vi "PXIe 4113 Update Channels.vi"(8 "error in (no error)":errorcluster, 10 "Array":dbl[](array[numeric]), 11 "Resource name in":refnum<k15>) -> (0 "error out":errorcluster, 3 "Resource name out":refnum<k15>)   [LabVIEW 2014, in "PXIe 4113 Engine.lvlib"]
uses:
  PXIe 4113 Engine.lvlib
  <instrlib>/niDCPower/nidcpower.llb/niDCPower Wait For Event - Event.ctl
  <vilib>/NI Veristand/Custom Device Tools/Custom Device Utility Library/Custom Device Utility Library.lvlib
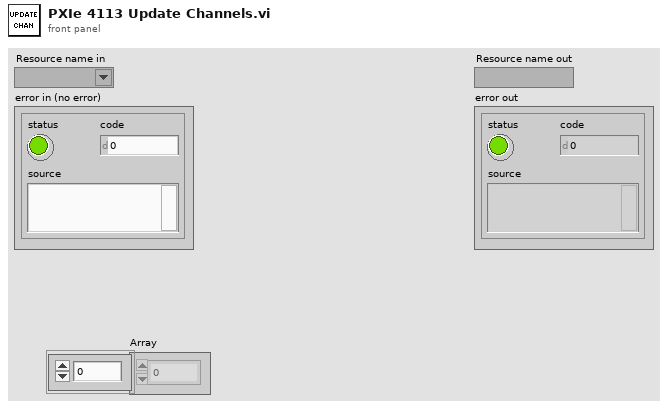
[diagram p1: front panel]
types:
  T1 = typedef "niDCPower Wait For Event - Event.ctl" = i32
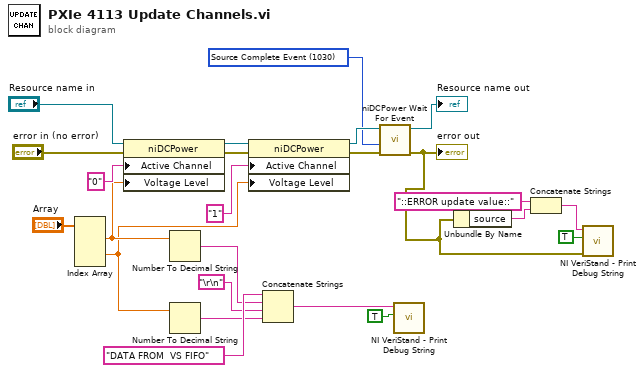
[diagram p0: block diagram]
diagram:
  w15 = T1 1030 items=["Source Complete Event"=1030, "Measure Complete Event"=1031, "Sequence Iteration Complete Event"=1032, "Sequence Engine Done Event"=1033, "Pulse Complete Event"=1051, "Ready For Pulse Trigger Event"=1052] ("event")
  n1 = Index Array(array="Array") -> (element #1=w10:dbl, element #3=w9:dbl)  [unwired: 4 in, 2 out]
  n2 = property class="niDCPower"(reference="Resource name in", error in="error in (no error)", "Active Channel"="0", "Voltage Level"=w10) -> (reference out=w20:refnum<k15>, error out=w19:errorcluster)
  n3 = Number To Decimal String(number=w10) -> (decimal integer string=w8:string)  [unwired: 1 in]
  n4 = Number To Decimal String(number=w9) -> (decimal integer string=w6:string)  [unwired: 1 in]
  n5 = property class="niDCPower"(reference=w20, error in=w19, "Active Channel"="1", "Voltage Level"=w9) -> (reference out=w17:refnum<k15>, error out=w16:errorcluster)
  n6 = Concatenate Strings("DATA FROM  VS FIFO" ("string"), w8, "\r\n", w6) -> (w11:string)
  n7 = call <instrlib>:"niDCPower Wait For Event.vi"("error in (no error)"=w16, "event"=w15, "instrument handle"=w17) -> ("error out"=w1:errorcluster, "instrument handle out"=→"Resource name out":refnum<k15>)  [unwired: 7 in]
  "error out" <- w1
  n8 = call <vilib>:"NI VeriStand - Print Debug String.vi"("Add to log file? (T)"=TRUE, "Message"=w11) -> ()  [unwired: 9 in, 1 out]
  n9 = Unbundle By Name(w1) -> ("source"=w4:string)
  n10 = Concatenate Strings("::ERROR update value::" ("string"), w4) -> (w5:string)
  n11 = call <vilib>:"NI VeriStand - Print Debug String.vi"("error in (no error)"=w1, "Add to log file? (T)"=TRUE, "Message"=w5) -> ()  [unwired: 8 in, 1 out]
